vi "CSM - Write INI String.vi"(5 "Section Name(\"\" as Default)":string, 7 "error in (no error)":errorcluster, 8 "String":string, 9 ">> Variable Name >>":string) -> (1 "error out":errorcluster, 2 "Key Replace?":bool)   [LabVIEW 2017, in "INI-Static-Variable-Support.lvlib"]
uses:
  INI-Static-Variable-Support.lvlib
  _Support/_fgv-oper.ctl
  _Support/global-csm-ini-db-change-flag.vi
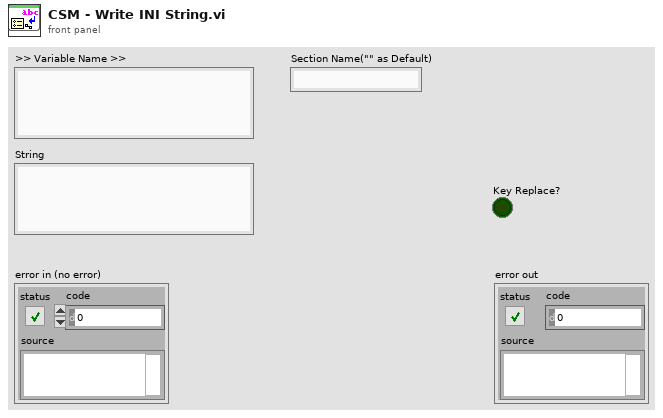
[diagram p1: front panel]
types:
  T1 = typedef "_fgv-oper.ctl" = enum16{"Read", "Write", "Sync"}
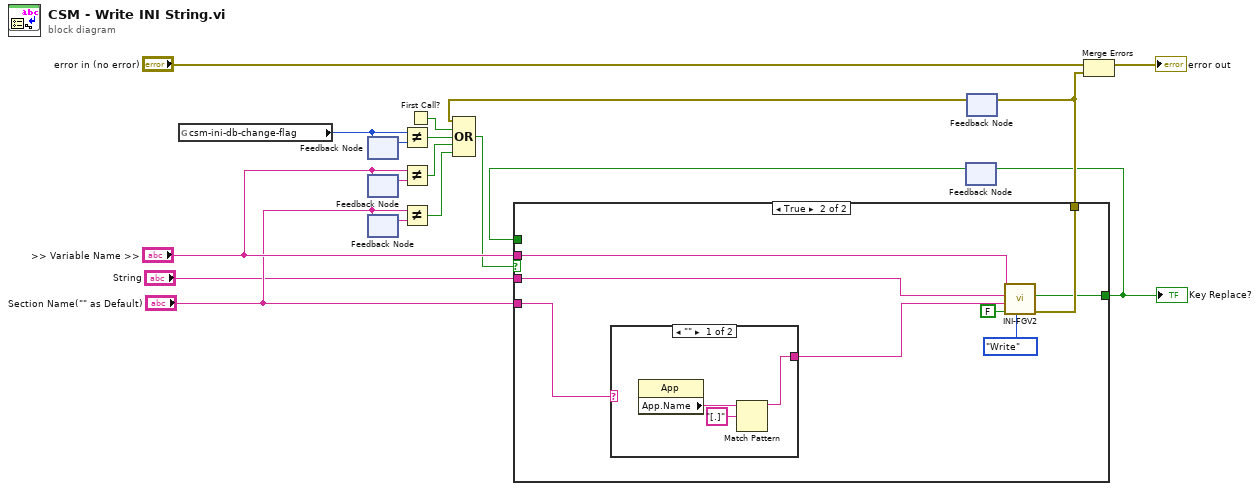
[diagram p0: block diagram]
diagram:
  n1 = global read "global-csm-ini-db-change-flag.vi" "csm-ini-db-change-flag"() -> (w16:u32)
  n2 = feedback #1() -> (w15:u32)  [unwired: 1 in]
  n3 = feedback-in #1(w16) -> ()
  n4 = feedback #2() -> (w12:string)  [unwired: 1 in]
  n5 = feedback-in #2(">> Variable Name >>") -> ()
  n6 = feedback #3() -> (w11:string)  [unwired: 1 in]
  n7 = feedback-in #3("Section Name(\"\" as Default)") -> ()
  n8 = Not Equal?(x=w16, y=w15) -> (x != y?=w14:bool)
  n9 = Not Equal?(x=">> Variable Name >>", y=w12) -> (x != y?=w8:bool)
  n10 = Not Equal?(x="Section Name(\"\" as Default)", y=w11) -> (x != y?=w7:bool)
  n11 = First Call?() -> (First Call?: T/F=w13:bool)
  n12 = feedback #4() -> (w4:bool)  [unwired: 1 in]
  n13 = feedback #5() -> (w3:errorcluster)  [unwired: 1 in]
  n14 = Compound Arithmetic op=OR(w3, w13, w14, w8, w7) -> (w2:bool)
  n15 = case shown="True" w2 {
    tunnel: [_ w25] -> w6
    tunnel: [w19 w24] -> w5
    tunnel: ">> Variable Name >>" -> [_ w23]
    tunnel: "Section Name(\"\" as Default)" -> [_ w22]
    tunnel: w4 -> [w19 _]
    tunnel: "String" -> [_ w20]
    frame False {
    }
    frame True {
      n16 = case shown="\"\"" w22 {
        selector: w22 -> [_ w31]
        tunnel: [w28 w31] -> w21
        frame "" {
          n17 = property class="App"() -> ("App.Name"=w29:string)  [unwired: 2 in, 2 out]
          n18 = Match Pattern(string=w29, regular expression="[.]") -> (before substring=w28:string)  [unwired: 1 in, 3 out]
        }
        frame Default {
        }
      }
      n19 = call "INI-FGV2.vi"("Enum"=_fgv-oper."Write", "Raw String? (F)"=FALSE, ">> Section >>"=w21, ">> Default Value >>"=w20, ">> Variable Name >>"=w23) -> ("error out"=w25:errorcluster, "Key?"=w24:bool)  [unwired: 4 in, 1 out]
    }
  }
  "Key Replace?" <- w5
  n20 = feedback-in #4(w5) -> ()
  n21 = feedback-in #5(w6) -> ()
  n22 = Merge Errors("error in (no error)", w6) -> (→"error out":errorcluster)
